vi "Read Range.vi"(11 "Interlock Bool in":refnum<class "Interlock Range.lvclass">) -> (1 "Exclude Range":bool, 2 "Range":cluster{"Upper Limit":dbl, "Lower Limit":dbl}, 3 "Interlock Bool out":refnum<class "Interlock Range.lvclass">)   [LabVIEW 2015, in "Interlocks.lvlib" / "Interlock Range.lvclass"]
uses:
  Interlock Range.lvclass
  Interlock Range.lvclass/Interlock Range.ctl
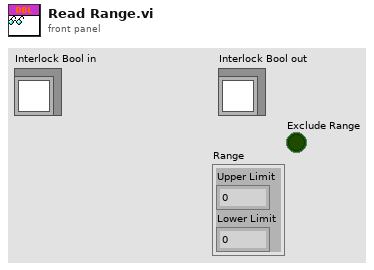
[diagram p1: front panel]
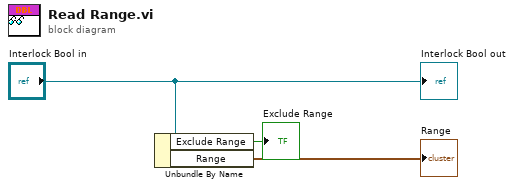
[diagram p0: block diagram]
diagram:
  n1 = Unbundle By Name("Interlock Bool in") -> ("Exclude Range"=→"Exclude Range":bool, "Range"=→"Range":cluster{"Upper Limit":dbl, "Lower Limit":dbl})
  "Interlock Bool out" <- "Interlock Bool in"
